vi "Automation VI.vi"() -> ()   [LabVIEW 2013]
panel:
  out "Tanque de Reserva":dbl
  out "Tanque de Almacenamiento":dbl
  out "Tanque de Reserva Vacio":bool
  out "Tanque de Almacenamiento Lleno":bool
  in  "Detener":bool
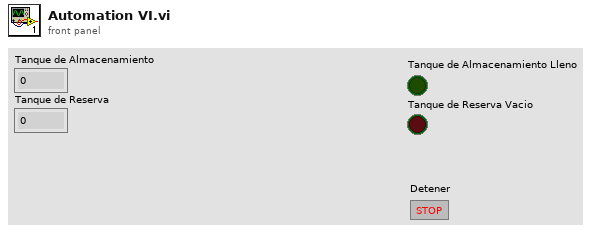
[diagram p1: front panel]
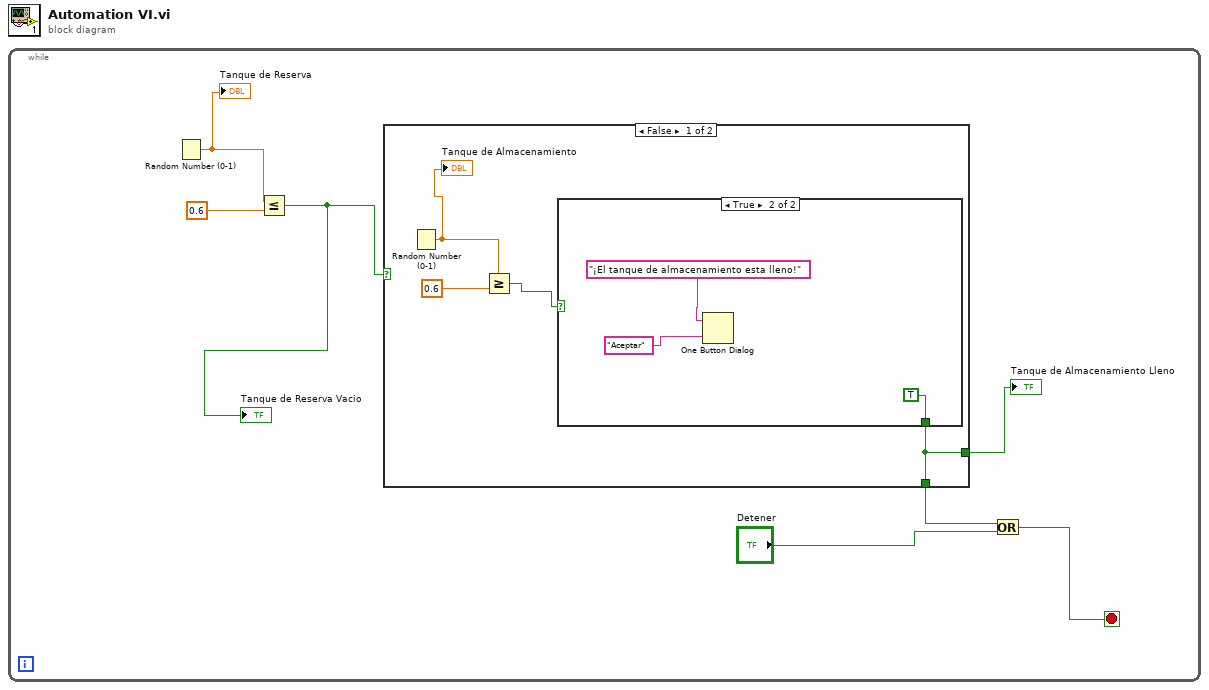
[diagram p0: block diagram]
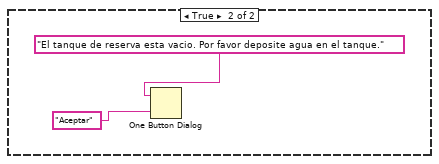
[diagram p3: hidden frame]
diagram:
  n1 = while {
    stop <- w4 stop-if-true
    n2 = Random Number (0-1)() -> (number: 0 to 1=w1:dbl)
    "Tanque de Reserva" <- w1
    n3 = Less Or Equal?(x=w1, y=0.6) -> (x <= y?=w3:bool)
    "Tanque de Reserva Vacio" <- w3
    n4 = case shown="False" w3 {
      tunnel: [w9 _] -> w6
      tunnel: [w9 _] -> w2
      frame False {
        n5 = Random Number (0-1)() -> (number: 0 to 1=w8:dbl)
        "Tanque de Almacenamiento" <- w8
        n6 = Greater Or Equal?(x=w8, y=0.6) -> (x >= y?=w10:bool)
        n7 = case shown="True" w10 {
          tunnel: [_ TRUE] -> w9
          frame False {
          }
          frame True {
            n8 = One Button Dialog(message="¡El tanque de almacenamiento esta lleno!", button name ("OK")="Aceptar") -> ()  [unwired: 1 out]
          }
        }
      }
      frame True {
        n9 = One Button Dialog(message="El tanque de reserva esta vacio. Por favor deposite agua en el tanque.", button name ("OK")="Aceptar") -> ()  [unwired: 1 out]
      }
    }
    "Tanque de Almacenamiento Lleno" <- w2
    n10 = Or(x=w6, y="Detener") -> (x .or. y?=w4:bool)
  }
